vi "AK Komm.vi"(6 "Aktionen":T2=enum."initialisieren", 11 "Daten":string[](array[string])) -> (0 "Verfügbare Gase":string[][](array[string]), 1 "Empfangsdaten":string[](array[string]), 2 "Error":T1, 3 "Status":string, 4 "Störung Kommunikation":bool, 5 "Konzentration":sgl, 7 "Betriebsart":string)   [LabVIEW 2020, in "Linearisierung v2.lvlib" / "Gasteiler.lvlib" / "AK Komm Gasteiler.lvlib"]
uses:
  AK Komm Gasteiler.lvlib
  Aktionen AK Komm.ctl
  Gasteiler Fehler.ctl
  Aktionen FGV Gasteiler Daten.ctl
  Gasteiler Type.ctl
  Gasteiler.lvlib
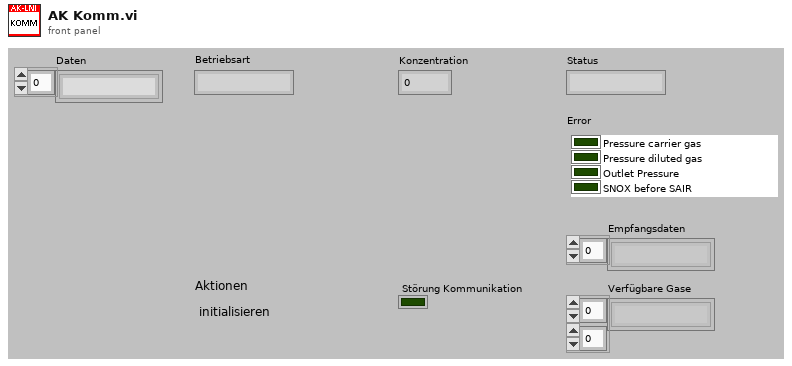
[diagram p1: front panel]
types:
  T1 = typedef "Linearisierung v2.lvlib/Gasteiler.lvlib/Gasteiler Fehler.ctl" = cluster{"Pressure carrier gas":bool, "Pressure diluted gas":bool, "Outlet Pressure":bool, "SNOX before SAIR":bool}
  T2 = typedef "Linearisierung v2.lvlib/Gasteiler.lvlib/AK Komm Gasteiler.lvlib/Aktionen AK Komm.ctl" = enum16{"lesen", "initialisieren", "beenden", "Status", "SMAN", "SREM", "STBY", "ASTF", "ASTZ", "SLST", "AGAT", "EGAK", "AGAK", "AKAK", "ADRU", "SKOP", "SVSA", "SVSZ", "SONO", "SAIR", "SNOX", "ANOX", "SSPL", "SRUC", "SLIN", "ALST", "ETYP", "SVIO", "LCYL", "CCYL", "DCYL", "SCYL", "GCYL", "DRGV", "DRDC"}
  T3 = typedef "Linearisierung v2.lvlib/Gasteiler.lvlib/Gasteiler Type.ctl" = enum16{"LNI Digital", "LNI Analoge", "AVL GDU ", "Horiba GDC", "HovaCal"}
  T4 = typedef "Linearisierung v2.lvlib/Gasteiler.lvlib/Aktionen FGV Gasteiler Daten.ctl" = enum16{"lesen", "Gasteiler Daten", "Seriellen Param.", "MB-Endwert", "laden", "speichern", "Anforderung", "TCP", "Aufzeichnung Start"}
  T5 = cluster{"Aktive":bool, "IP-Adresse":string, "Port":u16}
  T6 = typedef "Linearisierung v2.lvlib/GasteilerType.ctl" = u16
  T7 = typedef "AK-Schnittstelle.lvlib/AK Seriell.lvlib/Serielle Parameter.ctl" = cluster{"VISA resource name":refnum<visa-resource-name>, "baud rate":u32, "data bits":u16, "parity":u16, "stop bits":u16, "flow control":u16}
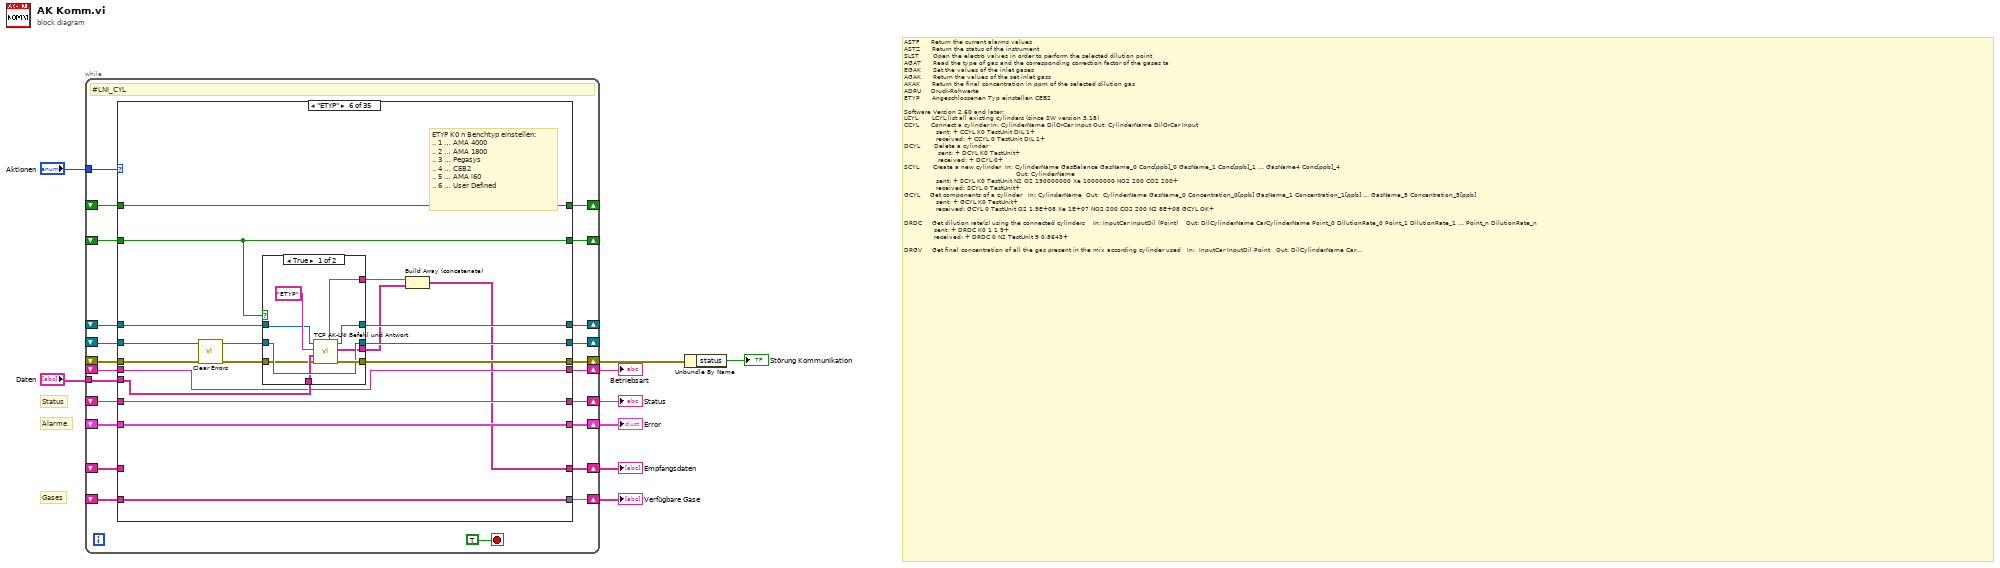
[diagram p0: block diagram]
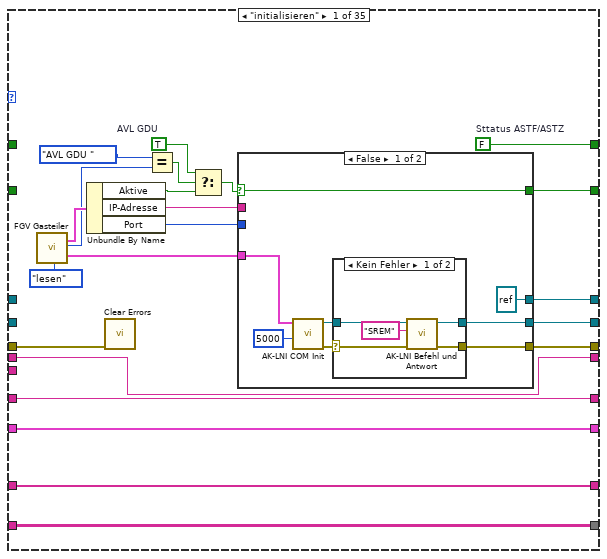
[diagram p2: hidden frame]
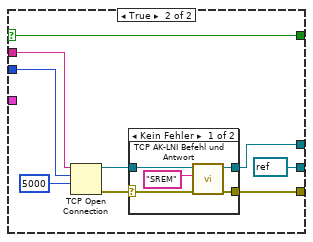
[diagram p4: hidden frame]
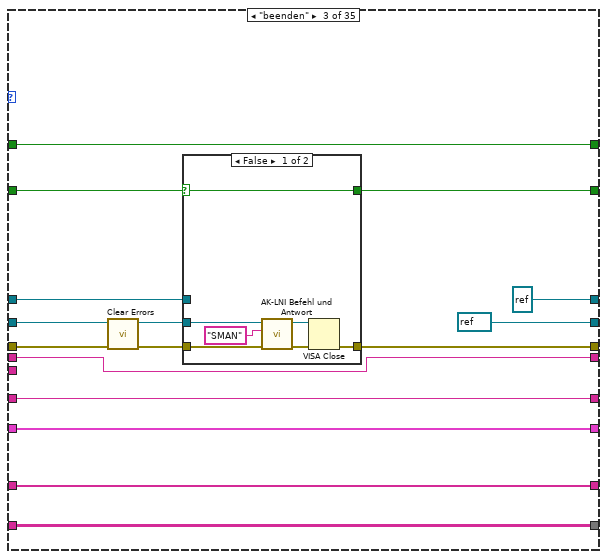
[diagram p7: hidden frame]
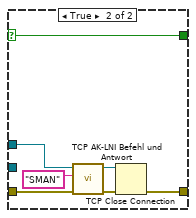
[diagram p8: hidden frame]
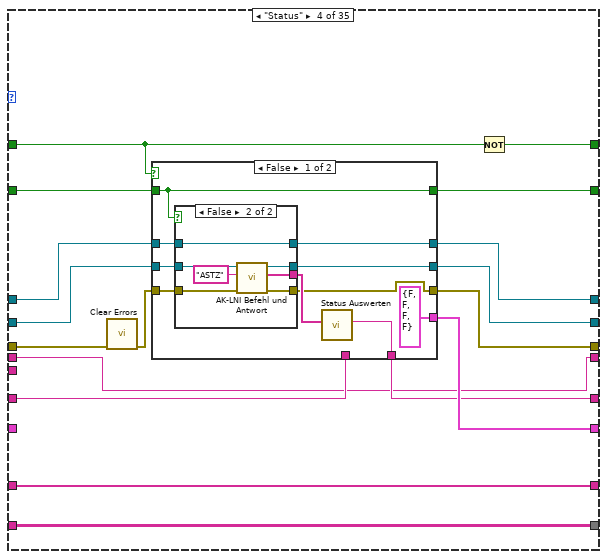
[diagram p9: hidden frame]
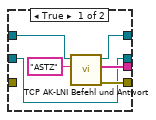
[diagram p10: hidden frame]
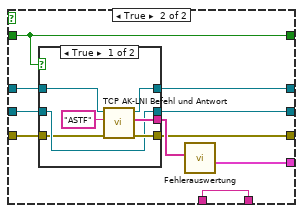
[diagram p11: hidden frame]
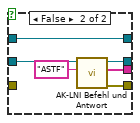
[diagram p12: hidden frame]
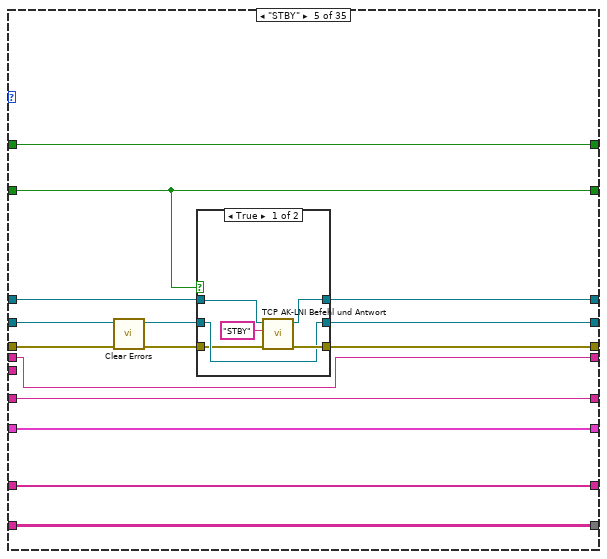
[diagram p13: hidden frame]
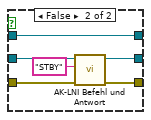
[diagram p14: hidden frame]
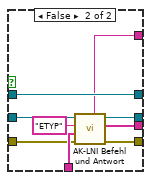
[diagram p15: hidden frame]
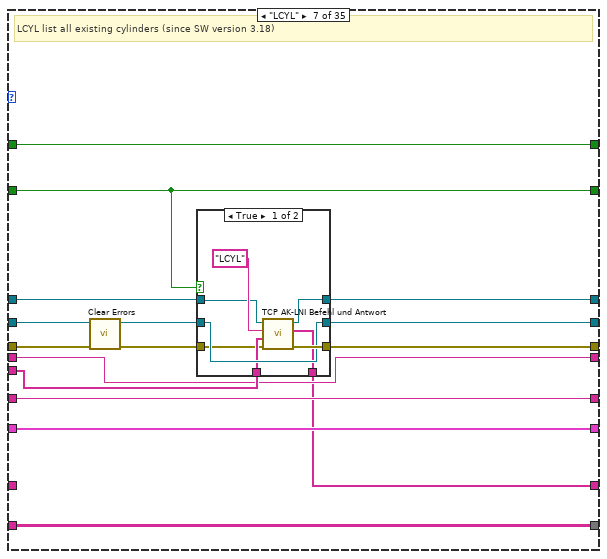
[diagram p16: hidden frame]
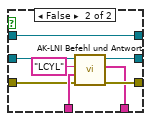
[diagram p17: hidden frame]
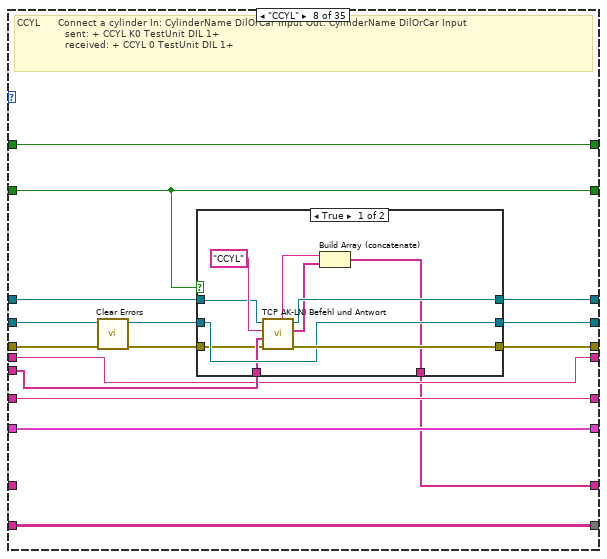
[diagram p18: hidden frame]
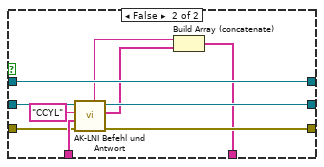
[diagram p19: hidden frame]
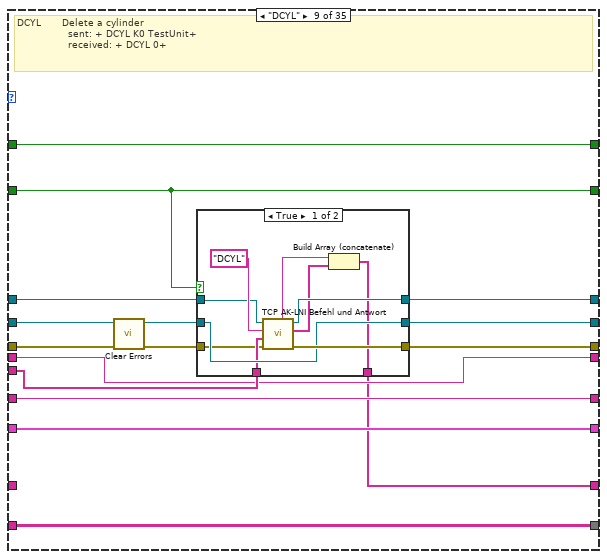
[diagram p20: hidden frame]
diagram:
  # "ASTF      Return the current alarms values\nASTZ      Return the status of the instrument \nSLST       Open the electro valves in order to perform the selected dilution point \nAGAT      Read the type of gas and the corresponding correction factor of the gases ta \nEGAK      Set the values of the inlet gases \nAGAK      Return the values of the set inlet gass \nAKAK      Return the final concentration in ppm of the selected dilution gas \nADRU     Druck-Rohwerte\nETYP      Angeschlossenen Typ einstellen CEB2\n\nSoftware Version 2.60 and later:\nLCYL       LCYL list all existing cylinders (since SW version 3.18)\nCCYL      Connect a cylinder In: CylinderName DilOrCar Input Out: CylinderName DilOrCar Input\n                sent: + CCYL K0 TestUnit DIL 1+\n                received: + CCYL 0 TestUnit DIL 1+\nDCYL       Delete a cylinder\n                 sent: + DCYL K0 TestUnit+\n                 received: + DCYL 0+\nSCYL       Create a new cylinder  In: CylinderName GasBalance GasName_0 Conc[ppb]_0 GasName_1 Conc[ppb]_1 … GasName4 Conc[ppb]_4\n                                                        Out: CylinderName\n                sent: + SCYL K0 TestUnit N2 O2 190000000 Xe 10000000 NO2 200 CO2 200+\n                received: SCYL 0 TestUnit+\nGCYL     Get components of a cylinder   In: CylinderName  Out:  CylinderName GasName_0 Concentration_0[ppb] GasName_1 Concentration_1[ppb] … GasName_5 Concentration_5[ppb]\n                sent: + GCYL K0 TestUnit+\n                received: GCYL 0 TestUnit O2 1.9E+08 Xe 1E+07 NO2 200 CO2 200 N2 8E+08 GCYL OK+\n\nDRDC     Get dilution rate(s) using the connected cylinders    In: InputCar InputDil (Point)    Out: DilCylinderName CarCylinderName Point_0 DilutionRate_0 Point_1 DilutionRate_1 … Point_n DilutionRate_n\n               sent: + DRDC K0 1 1 9+\n               received: + DRDC 0 N2 TestUnit 9 0.8643+\n\nDRGV     Get final concentration of all the gas present in the mix according cylinder used   In:  InputCar InputDil Point   Out: DilCylinderName CarCylinderName Point GasName_0 Concentration_0 GasName_1 Concentration_1 … GasName_n Concentration_n\n               sent: + DRGV K0 1 1 9+\n               received: + DRGV 0 N2 TestUnit 9 CO2 1.729 N2 9.983E+08 NO2 1.729 O2 1.642E+06 Xe 8.643E+04+ \n\nSKOP      Activate NOx converter tester \nSVSA      Open functions for the NOX converter tester \nSVSZ      Close functions for the NOX converter tester\nSONO     Open or close the valves in order to perform the NO phase\nSAIR       Open or close the valves in order to perform the Air phase of the NOx converter tester\nSNOX      Set the ozone in order to generate NO2 phase of the NOX converter tester (SONO and SAIR must have been sent previously)\nANOX      Read the set ozone value \n\n\n\nFür AVL\n\nSLIN        Um SLST senden zu können muss vorher SLIN gesendet werden\nALST        Abfrage Teilerstufe in %\n\nSVIO       Select the desired diluted inlet (if the option is installed). sent: + SVIO K0 13+ received: + SVIO 0"
  # "Gases"
  # "Status"
  # "Alarme"
  n1 = while {
    tunnel: "Aktionen" -> [w31]
    shift-right: [w30] -> _
    shift-left: _ -> [w29]
    shift-right: [w28] -> w4
    shift-left: _ -> [w27]
    shift-right: [w25] -> w7
    shift-left: _ -> [w26]
    tunnel: "Daten" -> [w24]
    shift-right: [w23] -> w5
    shift-left: _ -> [w22]
    shift-right: [w21] -> w6
    shift-left: _ -> [w20]
    shift-right: [w19] -> w3
    shift-left: _ -> [w18]
    shift-right: [w17] -> _
    shift-left: _ -> [w14]
    shift-right: [w16] -> _
    shift-left: _ -> [w15]
    shift-right: [w13] -> _
    shift-left: _ -> [w12]
    shift-right: [w11] -> w1
    shift-left: _ -> [w10]
    stop <- TRUE stop-if-true
    # "#LNI_CYL"
    n2 = case shown="\"ETYP\"" w31 {
      tunnel: [w49 w94 refnum<visa-resource-name> refnum ("VISA resource name") w140 w200 w229 w262 w293 w328 w363 w398 w433 w468 w504 w536 w567 w596 w626 w657 w694 w729 w767 w802 w834 w868 w899 w930 w963 w996 w1032 w1067 w1102 w1137 w1172 w1209] -> w30
      tunnel: w29 -> [_ w94 w104 w141 w201 w230 w263 w294 w329 w364 w399 w434 w469 w505 w537 w568 w597 w627 w658 w695 w730 w768 w803 w835 w869 w900 w931 w964 w997 w1033 w1068 w1103 w1138 w1173 w1210]
      tunnel: [w54 w95 w109 w131 w199 w228 w261 w292 w327 w362 w397 w432 w467 w503 w535 w561 w595 w625 w656 w693 w728 w766 w801 w833 w867 w898 w929 w962 w995 w1031 w1066 w1101 w1136 w1171 w1208] -> w28
      tunnel: w27 -> [w54 w95 w109 _ w199 w228 w261 w292 w327 w362 w397 w432 w467 w503 w535 _ w595 w625 w656 w693 w728 w766 w801 w833 w867 w898 w929 w962 w995 w1031 w1066 w1101 w1136 w1171 w1208]
      tunnel: w26 -> [w53 w92 w108 w129 w198 w227 w260 w291 w326 w361 w396 w431 w466 w502 w534 w565 _ _ w654 w691 w726 w764 w799 w832 w865 w896 w927 w960 w993 w1029 w1064 w1099 w1134 w1169 w1206]
      tunnel: [w53 w92 w108 w130 w198 w227 w260 w291 w326 w361 w396 w431 w466 w502 w534 w565 w593 w624 w654 w691 w726 w764 w799 w832 w865 w896 w927 w960 w993 w1029 w1064 w1099 w1134 w1169 w1206] -> w25
      tunnel: w24 -> [_ _ _ _ _ w219 w252 w283 w318 w353 w388 w423 w458 _ _ _ _ _ w655 w692 w727 w765 w800 _ w866 w897 w928 w961 w994 w1030 w1065 w1100 w1135 w1170 w1207]
      tunnel: [w51 w91 w106 w138 w196 w226 w259 w290 w325 w360 w395 w430 w465 w501 w533 w563 w591 w623 w653 w690 w725 w758 w798 w831 w864 w895 w926 w959 w992 w1028 w1063 w1098 w1133 w1168 w1205] -> w23
      tunnel: w22 -> [w51 w91 w106 w138 w196 w226 w259 w290 w325 w360 w395 w430 w465 w501 w533 w563 w591 w623 w653 w690 w725 _ w798 w831 w864 w895 w926 w959 w992 w1028 w1063 w1098 w1133 w1168 w1205]
      tunnel: [w52 w93 w107 w139 w197 w215 w250 w281 w316 w351 w386 w421 w456 w491 w523 w564 w592 w613 w645 w680 w715 w750 w787 w830 w856 w892 w918 w949 w984 w1019 w1053 w1088 w1123 w1158 w1193] -> w21
      tunnel: w20 -> [w52 w93 w107 w139 w197 _ _ _ _ _ _ _ _ _ _ w564 w592 _ _ _ _ _ _ _ _ _ _ _ _ _ _ _ _ _ _]
      tunnel: [w48 w90 w102 w137 w195 w225 w258 w289 w324 w359 w394 w429 w464 w500 w532 w562 w590 w622 w652 w689 w724 w761 w797 w829 w858 w894 w925 w958 w991 w1027 w1062 w1097 w1132 w1167 w1200] -> w19
      tunnel: w18 -> [w50 w90 w105 w136 w194 w224 w257 w288 w323 w358 w393 w428 w463 w499 w531 w560 w589 w621 w651 w688 w723 w760 w796 w828 w857 w893 w924 w957 w990 w1018 w1061 w1096 w1131 w1166 w1199]
      tunnel: [w44 w89 w101 w132 w193 w223 w256 w287 w322 w357 w392 w427 w462 w498 w530 w559 w588 w620 w650 w685 w722 w757 w795 w827 w855 w891 w923 w956 w989 w1026 w1060 w1095 w1130 w1165 w1198] -> w17
      tunnel: [w41 w88 refnum<k5> refnum ("Verbindungs-ID") w133 w191 w221 w254 w285 w320 w355 w390 w425 w460 w496 w528 w557 w586 w618 w648 w686 w720 w755 w793 w825 w853 w889 w921 w954 w987 w1024 w1058 w1093 w1128 w1163 w1196] -> w16
      tunnel: w15 -> [_ w88 w100 w134 w192 w222 w255 w286 w321 w356 w391 w426 w461 w497 w529 w558 w587 w619 w649 w687 w721 w756 w794 w826 w854 w890 w922 w955 w988 w1025 w1059 w1094 w1129 w1164 w1197]
      tunnel: w14 -> [_ w89 w103 w135 w193 w223 w256 w287 w322 w357 w392 w427 w462 w498 w530 w559 w588 w620 w650 w685 w722 w757 w795 w827 w855 w891 w923 w956 w989 w1026 w1060 w1095 w1130 w1165 w1198]
      tunnel: [w40 w87 w98 w127 w190 w220 w253 w284 w319 w354 w389 w424 w459 w495 w527 w556 w585 w617 w647 w684 w719 w754 w792 w824 w852 w888 w920 w953 w986 w1023 w1057 w1092 w1127 w1162 w1195] -> w13
      tunnel: w12 -> [_ w87 w98 w128 w190 w220 w253 w284 w319 w354 w389 w424 w459 w495 w527 w556 w585 w617 w647 w684 w719 w754 w792 w824 w852 w888 w920 w953 w986 w1023 w1057 w1092 w1127 w1162 w1195]
      tunnel: [w33 w86 w97 w126 w189 w218 w251 w282 w317 w352 w387 w422 w457 w494 w526 w555 w584 w616 w646 w683 w718 w753 w791 w823 w851 w887 w919 w952 w985 w1022 w1056 w1091 w1126 w1161 w1194] -> w11
      tunnel: w10 -> [w33 w86 w97 w126 w189 w218 w251 w282 w317 w352 w387 w422 w457 w494 w526 w555 _ w616 w646 w683 w718 w753 w791 w823 w851 w887 w919 w952 w985 w1022 w1056 w1091 w1126 w1161 w1194]
      frame "initialisieren" {
        w35 = TRUE  # AVL GDU
        w40 = FALSE  # Sttatus ASTF/ASTZ
        n3 = call "FGV Gasteiler.vi"("Aktionen"=Aktionen_FGV_Gasteiler_Daten."lesen") -> ("TCP"=w45:T5, "Gasteiler Type"=w39:T6, "Serielle Parameter"=w46:T7)  [unwired: 11 in, 5 out]
        n4 = Unbundle By Name(w45) -> ("Aktive"=w36:bool, "IP-Adresse"=w43:string, "Port"=w42:u16)
        n5 = call <vilib>:"Clear Errors.vi"("error in (no error)"=w50) -> ()  [unwired: 5 in, 2 out]
        n6 = Equal?(x=Gasteiler_Type."AVL GDU ", y=w39) -> (x = y?=w37:bool)
        n7 = Select(t=w35, s=w37, f=w36) -> (s? t:f=w34:bool)
        n8 = case shown="False" w34 {
          selector: w34 -> [w55 w78]
          tunnel: [w60 refnum<visa-resource-name> refnum ("VISA resource name")] -> w49
          tunnel: [w58 w73] -> w48
          tunnel: w46 -> [w57 _]
          tunnel: [w55 w78] -> w44
          tunnel: w43 -> [_ w76]
          tunnel: w42 -> [_ w75]
          tunnel: [refnum<k5> refnum ("connection ID") w70] -> w41
          frame False {
            n9 = call "AK-LNI COM Init.vi"("TimeOut (ms)"=u32 5000, "Schnittstelle"=w57) -> ("error out"=w59:errorcluster, "VISA resource name"=w61:refnum<visa-resource-name>)  [unwired: 8 in]
            n10 = case shown="Kein Fehler" w59 {
              selector: w59 -> [w64 w68]
              tunnel: w61 -> [w66 w69]
              tunnel: [w65 w69] -> w60
              tunnel: [w63 w68] -> w58
              frame No Error {
                n11 = call "AK-LNI Befehl und Antwort.vi"("Fehler (Eingang)"=w64, "Befehl (4 Zeichen)"="SREM", "VISA resource name"=w66) -> ("Fehler (Ausgang)"=w63:errorcluster, "VISA resource name out"=w65:refnum<visa-resource-name>)  [unwired: 3 in, 4 out]
              }
              frame Error {
              }
            }
          }
          frame True {
            n12 = TCP Open Connection(address=w76, remote port or service name=w75, timeout ms (60000)=5000 ("Timeout in ms (60000)")) -> (connection ID=w72:refnum<k5>, error out=w71:errorcluster)  [unwired: 2 in]
            n13 = case shown="Kein Fehler" w71 {
              selector: w71 -> [w79 w85]
              tunnel: [w83 w85] -> w73
              tunnel: w72 -> [w82 w84]
              tunnel: [w80 w84] -> w70
              frame No Error {
                n14 = call "TCP AK-LNI Befehl und Antwort.vi"("Fehler (Eingang)"=w79, "Befehl (4 Zeichen)"="SREM", "Verbindungs-ID"=w82) -> ("Fehler (Ausgang)"=w83:errorcluster, "Verbindungs-ID"=w80:refnum<k5>)  [unwired: 3 in, 4 out]
              }
              frame Error {
              }
            }
          }
        }
      }
      frame "lesen", Default {
      }
      frame "beenden" {
        n15 = call <vilib>:"Clear Errors.vi"("error in (no error)"=w105) -> ("error out"=w96:errorcluster)  [unwired: 5 in, 1 out]
        n16 = case shown="False" w103 {
          selector: w103 -> [w113 w124]
          tunnel: w104 -> [w117 _]
          tunnel: [w114 w119] -> w102
          tunnel: [w113 w124] -> w101
          tunnel: w100 -> [_ w123]
          tunnel: w96 -> [w111 w118]
          frame False {
            n17 = call "AK-LNI Befehl und Antwort.vi"("Fehler (Eingang)"=w111, "Befehl (4 Zeichen)"="SMAN", "VISA resource name"=w117) -> ("Fehler (Ausgang)"=w112:errorcluster, "VISA resource name out"=w115:refnum<visa-resource-name>)  [unwired: 3 in, 4 out]
            n18 = VISA Close(VISA resource name=w115, error in (no error)=w112) -> (error out=w114:errorcluster)
          }
          frame True {
            n19 = call "TCP AK-LNI Befehl und Antwort.vi"("Fehler (Eingang)"=w118, "Befehl (4 Zeichen)"="SMAN", "Verbindungs-ID"=w123) -> ("Fehler (Ausgang)"=w121:errorcluster, "Verbindungs-ID"=w120:refnum<k5>)  [unwired: 3 in, 4 out]
            n20 = TCP Close Connection(connection ID=w120, error in (no error)=w121) -> (error out=w119:errorcluster)  [unwired: 1 in, 1 out]
          }
        }
      }
      frame "Status" {
        n21 = call <vilib>:"Clear Errors.vi"("error in (no error)"=w136) -> ("error out"=w125:errorcluster)  [unwired: 5 in, 1 out]
        n22 = case shown="False" w128 {
          tunnel: w141 -> [w144 w174]
          tunnel: [w147 w173] -> w140
          tunnel: [w148 w171] -> w137
          tunnel: [T1 {"Pressure carrier gas"=FALSE, "Pressure diluted gas"=FALSE, "Outlet Pressure"=FALSE, "SNOX before SAIR"=FALSE} ("Error") w170] -> w131
          tunnel: w135 -> [w143 w167]
          tunnel: w134 -> [w145 w169]
          tunnel: [w146 w168] -> w133
          tunnel: [w143 w167] -> w132
          tunnel: [w150 w166] -> w130
          tunnel: w129 -> [_ w166]
          tunnel: w125 -> [w142 w165]
          frame False {
            n23 = case shown="False" w143 {
              tunnel: w144 -> [w154 w164]
              tunnel: [w154 w162] -> w147
              tunnel: [w156 w161] -> w151
              tunnel: [w155 w160] -> w148
              tunnel: w145 -> [w153 w159]
              tunnel: [w152 w159] -> w146
              tunnel: w142 -> [_ w158]
              frame True {
                n24 = call "TCP AK-LNI Befehl und Antwort.vi"("Befehl (4 Zeichen)"="ASTZ", "Verbindungs-ID"=w153) -> ("Fehler (Ausgang)"=w155:errorcluster, "Empfangsdaten"=w156:string[], "Verbindungs-ID"=w152:refnum<k5>)  [unwired: 4 in, 3 out]
              }
              frame False {
                n25 = call "AK-LNI Befehl und Antwort.vi"("Fehler (Eingang)"=w158, "Befehl (4 Zeichen)"="ASTZ", "VISA resource name"=w164) -> ("Fehler (Ausgang)"=w160:errorcluster, "Empfangsdaten"=w161:string[], "VISA resource name out"=w162:refnum<visa-resource-name>)  [unwired: 3 in, 3 out]
              }
            }
            n26 = call "Status Auswerten.vi"("Empfangsdaten"=w151) -> ("Status"=w150:string)  [unwired: 9 in, 1 out]
          }
          frame True {
            n27 = case shown="True" w167 {
              tunnel: w174 -> [w178 w187]
              tunnel: [w178 w185] -> w173
              tunnel: [w180 w184] -> w172
              tunnel: [w179 w183] -> w171
              tunnel: w169 -> [w177 w182]
              tunnel: [w176 w182] -> w168
              tunnel: w165 -> [w175 _]
              frame True {
                n28 = call "TCP AK-LNI Befehl und Antwort.vi"("Fehler (Eingang)"=w175, "Befehl (4 Zeichen)"="ASTF", "Verbindungs-ID"=w177) -> ("Fehler (Ausgang)"=w179:errorcluster, "Empfangsdaten"=w180:string[], "Verbindungs-ID"=w176:refnum<k5>)  [unwired: 3 in, 3 out]
              }
              frame False {
                n29 = call "AK-LNI Befehl und Antwort.vi"("Befehl (4 Zeichen)"="ASTF", "VISA resource name"=w187) -> ("Fehler (Ausgang)"=w183:errorcluster, "Empfangsdaten"=w184:string[], "VISA resource name out"=w185:refnum<visa-resource-name>)  [unwired: 4 in, 3 out]
              }
            }
            n30 = call "Fehlerauswertung.vi"("Empfangsdaten"=w172) -> ("Error"=w170:T1)  [unwired: 9 in, 1 out]
          }
        }
        n31 = Not(x=w128) -> (.not. x?=w127:bool)
      }
      frame "STBY" {
        n32 = call <vilib>:"Clear Errors.vi"("error in (no error)"=w194) -> ("error out"=w188:errorcluster)  [unwired: 5 in, 1 out]
        n33 = case shown="True" w193 {
          tunnel: w201 -> [w204 w213]
          tunnel: [w204 w211] -> w200
          tunnel: [w206 w210] -> w195
          tunnel: w192 -> [w205 w209]
          tunnel: [w203 w209] -> w191
          tunnel: w188 -> [w202 w208]
          frame True {
            n34 = call "TCP AK-LNI Befehl und Antwort.vi"("Fehler (Eingang)"=w202, "Befehl (4 Zeichen)"="STBY", "Verbindungs-ID"=w205) -> ("Fehler (Ausgang)"=w206:errorcluster, "Verbindungs-ID"=w203:refnum<k5>)  [unwired: 3 in, 4 out]
          }
          frame False {
            n35 = call "AK-LNI Befehl und Antwort.vi"("Fehler (Eingang)"=w208, "Befehl (4 Zeichen)"="STBY", "VISA resource name"=w213) -> ("Fehler (Ausgang)"=w210:errorcluster, "VISA resource name out"=w211:refnum<visa-resource-name>)  [unwired: 3 in, 4 out]
          }
        }
      }
      frame "ETYP" {
        # "ETYP K0 n Benchtyp einstellen:\n.. 1 … AMA 4000\n.. 2 … AMA 1800\n.. 3 … Pegasys\n.. 4 … CEB2\n.. 5 … AMA i60\n.. 6 … User Defined"
        n36 = call <vilib>:"Clear Errors.vi"("error in (no error)"=w224) -> ("error out"=w214:errorcluster)  [unwired: 5 in, 1 out]
        n37 = case shown="True" w223 {
          tunnel: w230 -> [w236 w248]
          tunnel: [w236 w246] -> w229
          tunnel: [w238 w245] -> w225
          tunnel: w222 -> [w237 w244]
          tunnel: [w235 w244] -> w221
          tunnel: w219 -> [w234 w243]
          tunnel: [w233 w242] -> w217
          tunnel: [w232 w241] -> w216
          tunnel: w214 -> [w231 w240]
          frame True {
            n38 = call "TCP AK-LNI Befehl und Antwort.vi"("Fehler (Eingang)"=w231, "Sendedaten"=w234, "Befehl (4 Zeichen)"="ETYP", "Verbindungs-ID"=w237) -> ("Fehler (Ausgang)"=w238:errorcluster, "Empfangsdaten"=w233:string[], "Verbindungs-ID"=w235:refnum<k5>, "Befehl (Antwort)"=w232:string)  [unwired: 2 in, 2 out]
          }
          frame False {
            n39 = call "AK-LNI Befehl und Antwort.vi"("Fehler (Eingang)"=w240, "Sendedaten"=w243, "Befehl (4 Zeichen)"="ETYP", "VISA resource name"=w248) -> ("Fehler (Ausgang)"=w245:errorcluster, "Empfangsdaten"=w242:string[], "VISA resource name out"=w246:refnum<visa-resource-name>, "Befehl (Antwort)"=w241:string)  [unwired: 2 in, 2 out]
          }
        }
        n40 = Build Array (concatenate)(w216, w217) -> (w215:string[])
      }
      frame "LCYL" {
        # "LCYL list all existing cylinders (since SW version 3.18)"
        n41 = call <vilib>:"Clear Errors.vi"("error in (no error)"=w257) -> ("error out"=w249:errorcluster)  [unwired: 5 in, 1 out]
        n42 = case shown="True" w256 {
          tunnel: w263 -> [w268 w279]
          tunnel: [w268 w277] -> w262
          tunnel: [w270 w276] -> w258
          tunnel: w255 -> [w269 w275]
          tunnel: [w267 w275] -> w254
          tunnel: w252 -> [w266 w274]
          tunnel: [w265 w273] -> w250
          tunnel: w249 -> [w264 w272]
          frame True {
            n43 = call "TCP AK-LNI Befehl und Antwort.vi"("Fehler (Eingang)"=w264, "Sendedaten"=w266, "Befehl (4 Zeichen)"="LCYL", "Verbindungs-ID"=w269) -> ("Fehler (Ausgang)"=w270:errorcluster, "Empfangsdaten"=w265:string[], "Verbindungs-ID"=w267:refnum<k5>)  [unwired: 2 in, 3 out]
          }
          frame False {
            n44 = call "AK-LNI Befehl und Antwort.vi"("Fehler (Eingang)"=w272, "Sendedaten"=w274, "Befehl (4 Zeichen)"="LCYL", "VISA resource name"=w279) -> ("Fehler (Ausgang)"=w276:errorcluster, "Empfangsdaten"=w273:string[], "VISA resource name out"=w277:refnum<visa-resource-name>)  [unwired: 2 in, 3 out]
          }
        }
      }
      frame "CCYL" {
        # "CCYL      Connect a cylinder In: CylinderName DilOrCar Input Out: CylinderName DilOrCar Input\n                sent: + CCYL K0 TestUnit DIL 1+\n                received: + CCYL 0 TestUnit DIL 1+"
        n45 = call <vilib>:"Clear Errors.vi"("error in (no error)"=w288) -> ("error out"=w280:errorcluster)  [unwired: 5 in, 1 out]
        n46 = case shown="True" w287 {
          tunnel: w294 -> [w301 w314]
          tunnel: [w301 w312] -> w293
          tunnel: [w303 w311] -> w289
          tunnel: w286 -> [w302 w310]
          tunnel: [w300 w310] -> w285
          tunnel: w283 -> [w299 w309]
          tunnel: [w296 w306] -> w281
          tunnel: w280 -> [w295 w305]
          frame True {
            n47 = call "TCP AK-LNI Befehl und Antwort.vi"("Fehler (Eingang)"=w295, "Sendedaten"=w299, "Befehl (4 Zeichen)"="CCYL", "Verbindungs-ID"=w302) -> ("Fehler (Ausgang)"=w303:errorcluster, "Empfangsdaten"=w297:string[], "Verbindungs-ID"=w300:refnum<k5>, "Befehl (Antwort)"=w298:string)  [unwired: 2 in, 2 out]
            n48 = Build Array (concatenate)(w298, w297) -> (w296:string[])
          }
          frame False {
            n49 = call "AK-LNI Befehl und Antwort.vi"("Fehler (Eingang)"=w305, "Sendedaten"=w309, "Befehl (4 Zeichen)"="CCYL", "VISA resource name"=w314) -> ("Fehler (Ausgang)"=w311:errorcluster, "Empfangsdaten"=w307:string[], "VISA resource name out"=w312:refnum<visa-resource-name>, "Befehl (Antwort)"=w308:string)  [unwired: 2 in, 2 out]
            n50 = Build Array (concatenate)(w308, w307) -> (w306:string[])
          }
        }
      }
      frame "DCYL" {
        # "DCYL       Delete a cylinder\n                 sent: + DCYL K0 TestUnit+\n                 received: + DCYL 0+"
        n51 = call <vilib>:"Clear Errors.vi"("error in (no error)"=w323) -> ("error out"=w315:errorcluster)  [unwired: 5 in, 1 out]
        n52 = case shown="True" w322 {
          tunnel: w329 -> [w336 w349]
          tunnel: [w336 w347] -> w328
          tunnel: [w338 w346] -> w324
          tunnel: w321 -> [w337 w345]
          tunnel: [w335 w345] -> w320
          tunnel: w318 -> [w334 w344]
          tunnel: [w331 w341] -> w316
          tunnel: w315 -> [w330 w340]
          frame True {
            n53 = call "TCP AK-LNI Befehl und Antwort.vi"("Fehler (Eingang)"=w330, "Sendedaten"=w334, "Befehl (4 Zeichen)"="DCYL", "Verbindungs-ID"=w337) -> ("Fehler (Ausgang)"=w338:errorcluster, "Empfangsdaten"=w332:string[], "Verbindungs-ID"=w335:refnum<k5>, "Befehl (Antwort)"=w333:string)  [unwired: 2 in, 2 out]
            n54 = Build Array (concatenate)(w333, w332) -> (w331:string[])
          }
          frame False {
            n55 = call "AK-LNI Befehl und Antwort.vi"("Fehler (Eingang)"=w340, "Sendedaten"=w344, "Befehl (4 Zeichen)"="DCYL", "VISA resource name"=w349) -> ("Fehler (Ausgang)"=w346:errorcluster, "Empfangsdaten"=w342:string[], "VISA resource name out"=w347:refnum<visa-resource-name>, "Befehl (Antwort)"=w343:string)  [unwired: 2 in, 2 out]
            n56 = Build Array (concatenate)(w343, w342) -> (w341:string[])
          }
        }
      }
      frame "SCYL" {
        # "SCYL       Create a new cylinder  In: CylinderName GasBalance GasName_0 Conc[ppb]_0 GasName_1 Conc[ppb]_1 … GasName4 Conc[ppb]_4\n                                                        Out: CylinderName\n                sent: + SCYL K0 TestUnit N2 O2 190000000 Xe 10000000 NO2 200 CO2 200+\n                received: SCYL 0 TestUnit+"
        n57 = call <vilib>:"Clear Errors.vi"("error in (no error)"=w358) -> ("error out"=w350:errorcluster)  [unwired: 5 in, 1 out]
        n58 = case shown="True" w357 {
          tunnel: w364 -> [w371 w384]
          tunnel: [w371 w382] -> w363
          tunnel: [w373 w381] -> w359
          tunnel: w356 -> [w372 w380]
          tunnel: [w370 w380] -> w355
          tunnel: w353 -> [w369 w379]
          tunnel: [w366 w376] -> w351
          tunnel: w350 -> [w365 w375]
          frame True {
            n59 = call "TCP AK-LNI Befehl und Antwort.vi"("Fehler (Eingang)"=w365, "Sendedaten"=w369, "Befehl (4 Zeichen)"="SCYL", "Verbindungs-ID"=w372) -> ("Fehler (Ausgang)"=w373:errorcluster, "Empfangsdaten"=w367:string[], "Verbindungs-ID"=w370:refnum<k5>, "Befehl (Antwort)"=w368:string)  [unwired: 2 in, 2 out]
            n60 = Build Array (concatenate)(w368, w367) -> (w366:string[])
          }
          frame False {
            n61 = call "AK-LNI Befehl und Antwort.vi"("Fehler (Eingang)"=w375, "Sendedaten"=w379, "Befehl (4 Zeichen)"="SCYL", "VISA resource name"=w384) -> ("Fehler (Ausgang)"=w381:errorcluster, "Empfangsdaten"=w377:string[], "VISA resource name out"=w382:refnum<visa-resource-name>, "Befehl (Antwort)"=w378:string)  [unwired: 2 in, 2 out]
            n62 = Build Array (concatenate)(w378, w377) -> (w376:string[])
          }
        }
      }
      frame "GCYL" {
        # "GCYL     Get components of a cylinder   In: CylinderName  Out:  CylinderName GasName_0 Concentration_0[ppb] GasName_1 Concentration_1[ppb] … GasName_5 Concentration_5[ppb]\n                sent: + GCYL K0 TestUnit+\n                received: GCYL 0 TestUnit O2 1.9E+08 Xe 1E+07 NO2 200 CO2 200 N2 8E+08 GCYL OK+"
        n63 = call <vilib>:"Clear Errors.vi"("error in (no error)"=w393) -> ("error out"=w385:errorcluster)  [unwired: 5 in, 1 out]
        n64 = case shown="True" w392 {
          tunnel: w399 -> [w406 w419]
          tunnel: [w406 w417] -> w398
          tunnel: [w408 w416] -> w394
          tunnel: w391 -> [w407 w415]
          tunnel: [w405 w415] -> w390
          tunnel: w388 -> [w404 w414]
          tunnel: [w401 w411] -> w386
          tunnel: w385 -> [w400 w410]
          frame True {
            n65 = call "TCP AK-LNI Befehl und Antwort.vi"("Fehler (Eingang)"=w400, "Sendedaten"=w404, "Befehl (4 Zeichen)"="GCYL", "Verbindungs-ID"=w407) -> ("Fehler (Ausgang)"=w408:errorcluster, "Empfangsdaten"=w402:string[], "Verbindungs-ID"=w405:refnum<k5>, "Befehl (Antwort)"=w403:string)  [unwired: 2 in, 2 out]
            n66 = Build Array (concatenate)(w403, w402) -> (w401:string[])
          }
          frame False {
            n67 = call "AK-LNI Befehl und Antwort.vi"("Fehler (Eingang)"=w410, "Sendedaten"=w414, "Befehl (4 Zeichen)"="GCYL", "VISA resource name"=w419) -> ("Fehler (Ausgang)"=w416:errorcluster, "Empfangsdaten"=w412:string[], "VISA resource name out"=w417:refnum<visa-resource-name>, "Befehl (Antwort)"=w413:string)  [unwired: 2 in, 2 out]
            n68 = Build Array (concatenate)(w413, w412) -> (w411:string[])
          }
        }
      }
      frame "DRGV" {
        # "Get final concentration of all the gas present in the mix according cylinder used   In:  InputCar InputDil Point   Out: DilCylinderName CarCylinderName Point GasName_0 Concentration_0 GasName_1 Concentration_1 … GasName_n Concentration_n\n               sent: + DRGV K0 1 1 9+\n               received: + DRGV 0 N2 TestUnit 9 CO2 1.729 N2 9.983E+08 NO2 1.729 O2 1.642E+06 Xe 8.643E+04+"
        n69 = call <vilib>:"Clear Errors.vi"("error in (no error)"=w428) -> ("error out"=w420:errorcluster)  [unwired: 5 in, 1 out]
        n70 = case shown="True" w427 {
          tunnel: w434 -> [w441 w454]
          tunnel: [w441 w452] -> w433
          tunnel: [w443 w451] -> w429
          tunnel: w426 -> [w442 w450]
          tunnel: [w440 w450] -> w425
          tunnel: w423 -> [w439 w449]
          tunnel: [w436 w446] -> w421
          tunnel: w420 -> [w435 w445]
          frame True {
            n71 = call "TCP AK-LNI Befehl und Antwort.vi"("Fehler (Eingang)"=w435, "Sendedaten"=w439, "Befehl (4 Zeichen)"="DRGV", "Verbindungs-ID"=w442) -> ("Fehler (Ausgang)"=w443:errorcluster, "Empfangsdaten"=w437:string[], "Verbindungs-ID"=w440:refnum<k5>, "Befehl (Antwort)"=w438:string)  [unwired: 2 in, 2 out]
            n72 = Build Array (concatenate)(w438, w437) -> (w436:string[])
          }
          frame False {
            n73 = call "AK-LNI Befehl und Antwort.vi"("Fehler (Eingang)"=w445, "Sendedaten"=w449, "Befehl (4 Zeichen)"="DRGV", "VISA resource name"=w454) -> ("Fehler (Ausgang)"=w451:errorcluster, "Empfangsdaten"=w447:string[], "VISA resource name out"=w452:refnum<visa-resource-name>, "Befehl (Antwort)"=w448:string)  [unwired: 2 in, 2 out]
            n74 = Build Array (concatenate)(w448, w447) -> (w446:string[])
          }
        }
      }
      frame "DRDC" {
        # "Get dilution rate(s) using the connected cylinders    In: InputCar InputDil (Point)    Out: DilCylinderName CarCylinderName Point_0 DilutionRate_0 Point_1 DilutionRate_1 … Point_n DilutionRate_n\n               sent: + DRDC K0 1 1 9+\n               received: + DRDC 0 N2 TestUnit 9 0.8643+"
        n75 = call <vilib>:"Clear Errors.vi"("error in (no error)"=w463) -> ("error out"=w455:errorcluster)  [unwired: 5 in, 1 out]
        n76 = case shown="True" w462 {
          tunnel: w469 -> [w476 w489]
          tunnel: [w476 w487] -> w468
          tunnel: [w478 w486] -> w464
          tunnel: w461 -> [w477 w485]
          tunnel: [w475 w485] -> w460
          tunnel: w458 -> [w474 w484]
          tunnel: [w471 w481] -> w456
          tunnel: w455 -> [w470 w480]
          frame True {
            n77 = call "TCP AK-LNI Befehl und Antwort.vi"("Fehler (Eingang)"=w470, "Sendedaten"=w474, "Befehl (4 Zeichen)"="DRDC", "Verbindungs-ID"=w477) -> ("Fehler (Ausgang)"=w478:errorcluster, "Empfangsdaten"=w472:string[], "Verbindungs-ID"=w475:refnum<k5>, "Befehl (Antwort)"=w473:string)  [unwired: 2 in, 2 out]
            n78 = Build Array (concatenate)(w473, w472) -> (w471:string[])
          }
          frame False {
            n79 = call "AK-LNI Befehl und Antwort.vi"("Fehler (Eingang)"=w480, "Sendedaten"=w484, "Befehl (4 Zeichen)"="DRDC", "VISA resource name"=w489) -> ("Fehler (Ausgang)"=w486:errorcluster, "Empfangsdaten"=w482:string[], "VISA resource name out"=w487:refnum<visa-resource-name>, "Befehl (Antwort)"=w483:string)  [unwired: 2 in, 2 out]
            n80 = Build Array (concatenate)(w483, w482) -> (w481:string[])
          }
        }
      }
      frame "SMAN" {
        n81 = call <vilib>:"Clear Errors.vi"("error in (no error)"=w499) -> ("error out"=w490:errorcluster)  [unwired: 5 in, 1 out]
        n82 = case shown="False" w498 {
          tunnel: w505 -> [w511 w521]
          tunnel: [w511 w519] -> w504
          tunnel: [w512 w518] -> w500
          tunnel: w497 -> [w510 w517]
          tunnel: [w509 w517] -> w496
          tunnel: [w508 w516] -> w492
          tunnel: [w507 w515] -> w493
          tunnel: w490 -> [w506 w514]
          frame True {
            n83 = call "TCP AK-LNI Befehl und Antwort.vi"("Fehler (Eingang)"=w506, "Befehl (4 Zeichen)"="SMAN", "Verbindungs-ID"=w510) -> ("Fehler (Ausgang)"=w512:errorcluster, "Empfangsdaten"=w508:string[], "Verbindungs-ID"=w509:refnum<k5>, "Befehl (Antwort)"=w507:string)  [unwired: 3 in, 2 out]
          }
          frame False {
            n84 = call "AK-LNI Befehl und Antwort.vi"("Fehler (Eingang)"=w514, "Befehl (4 Zeichen)"="SMAN", "VISA resource name"=w521) -> ("Fehler (Ausgang)"=w518:errorcluster, "Empfangsdaten"=w516:string[], "VISA resource name out"=w519:refnum<visa-resource-name>, "Befehl (Antwort)"=w515:string)  [unwired: 3 in, 2 out]
          }
        }
        n85 = Build Array (concatenate)(w493, w492) -> (w491:string[])
      }
      frame "SREM" {
        n86 = call <vilib>:"Clear Errors.vi"("error in (no error)"=w531) -> ("error out"=w522:errorcluster)  [unwired: 5 in, 1 out]
        n87 = case shown="False" w530 {
          tunnel: w537 -> [w541 w553]
          tunnel: [w541 w551] -> w536
          tunnel: [w544 w550] -> w532
          tunnel: w529 -> [w543 w549]
          tunnel: [w542 w549] -> w528
          tunnel: [w540 w548] -> w524
          tunnel: [w539 w546] -> w525
          tunnel: w522 -> [w538 w547]
          frame True {
            n88 = call "TCP AK-LNI Befehl und Antwort.vi"("Fehler (Eingang)"=w538, "Befehl (4 Zeichen)"="SREM", "Verbindungs-ID"=w543) -> ("Fehler (Ausgang)"=w544:errorcluster, "Empfangsdaten"=w540:string[], "Verbindungs-ID"=w542:refnum<k5>, "Befehl (Antwort)"=w539:string)  [unwired: 3 in, 2 out]
          }
          frame False {
            n89 = call "AK-LNI Befehl und Antwort.vi"("Fehler (Eingang)"=w547, "Befehl (4 Zeichen)"="SREM", "VISA resource name"=w553) -> ("Fehler (Ausgang)"=w550:errorcluster, "Empfangsdaten"=w548:string[], "VISA resource name out"=w551:refnum<visa-resource-name>, "Befehl (Antwort)"=w546:string)  [unwired: 3 in, 2 out]
          }
        }
        n90 = Build Array (concatenate)(w525, w524) -> (w523:string[])
      }
      frame "ASTF" {
        # "Return the current alarms values\n\nBefehl:     ASTF K0\nAntwort:  ASTF ES X Y ... N\n\nAlarm Code: 0  if there are no alarms\n                     1  if the pressure of the carrier gas is out of range\n                     2  if the pressure of the diluted gas is out of range\n                     3  if the outlet pressure is out of range\n                     4  if the command SNOX have been sent before the SAIR command"
        n91 = call <vilib>:"Clear Errors.vi"("error in (no error)"=w560) -> ("error out"=w554:errorcluster)  [unwired: 5 in, 1 out]
        n92 = case shown="True" w559 {
          tunnel: w568 -> [w572 w582]
          tunnel: [w572 w580] -> w567
          tunnel: [w574 w579] -> w566
          tunnel: [w573 w578] -> w562
          tunnel: w558 -> [w571 w577]
          tunnel: [w570 w577] -> w557
          tunnel: w554 -> [w569 w576]
          frame True {
            n93 = call "TCP AK-LNI Befehl und Antwort.vi"("Fehler (Eingang)"=w569, "Befehl (4 Zeichen)"="ASTF", "Verbindungs-ID"=w571) -> ("Fehler (Ausgang)"=w573:errorcluster, "Empfangsdaten"=w574:string[], "Verbindungs-ID"=w570:refnum<k5>)  [unwired: 3 in, 3 out]
          }
          frame False {
            n94 = call "AK-LNI Befehl und Antwort.vi"("Fehler (Eingang)"=w576, "Befehl (4 Zeichen)"="ASTF", "VISA resource name"=w582) -> ("Fehler (Ausgang)"=w578:errorcluster, "Empfangsdaten"=w579:string[], "VISA resource name out"=w580:refnum<visa-resource-name>)  [unwired: 3 in, 3 out]
          }
        }
        n95 = call "Fehlerauswertung.vi"("Empfangsdaten"=w566) -> ("Error"=w561:T1)  [unwired: 9 in, 1 out]
      }
      frame "ASTZ" {
        # "Return the status of the instrument \n\nBefehl:     ASTZ K0\nAntwort:  ASTZ ES Stat1 Stat2\n\nStat1 = SREM oder SMAN\nStat2 = STBY\n             SLST Point\n             SSPL Phase\n             SRUC Phase\n             SAIR\n             SONO\n             SNOX O3_Value"
        n96 = call <vilib>:"Clear Errors.vi"("error in (no error)"=w589) -> ("error out"=w583:errorcluster)  [unwired: 5 in, 1 out]
        n97 = case shown="True" w588 {
          tunnel: w597 -> [w601 w611]
          tunnel: [w601 w609] -> w596
          tunnel: [w603 w608] -> w594
          tunnel: [w602 w607] -> w590
          tunnel: w587 -> [w600 w606]
          tunnel: [w599 w606] -> w586
          tunnel: w583 -> [w598 w605]
          frame True {
            n98 = call "TCP AK-LNI Befehl und Antwort.vi"("Fehler (Eingang)"=w598, "Befehl (4 Zeichen)"="ASTZ", "Verbindungs-ID"=w600) -> ("Fehler (Ausgang)"=w602:errorcluster, "Empfangsdaten"=w603:string[], "Verbindungs-ID"=w599:refnum<k5>)  [unwired: 3 in, 3 out]
          }
          frame False {
            n99 = call "AK-LNI Befehl und Antwort.vi"("Fehler (Eingang)"=w605, "Befehl (4 Zeichen)"="ASTZ", "VISA resource name"=w611) -> ("Fehler (Ausgang)"=w607:errorcluster, "Empfangsdaten"=w608:string[], "VISA resource name out"=w609:refnum<visa-resource-name>)  [unwired: 3 in, 3 out]
          }
        }
        n100 = call "Status Auswerten.vi"("Empfangsdaten"=w594) -> ("Status"=w593:string, "Betriebsart"=w584:string)  [unwired: 9 in]
      }
      frame "SLIN" {
        n101 = call <vilib>:"Clear Errors.vi"("error in (no error)"=w621) -> ("error out"=w612:errorcluster)  [unwired: 5 in, 1 out]
        n102 = case shown="False" w620 {
          tunnel: w627 -> [w632 w643]
          tunnel: [w632 w641] -> w626
          tunnel: [w634 w640] -> w614
          tunnel: [w633 w639] -> w622
          tunnel: w619 -> [w631 w638]
          tunnel: [w630 w638] -> w618
          tunnel: [w629 w637] -> w615
          tunnel: w612 -> [w628 w636]
          frame True {
            n103 = call "TCP AK-LNI Befehl und Antwort.vi"("Fehler (Eingang)"=w628, "Befehl (4 Zeichen)"="SLIN", "Verbindungs-ID"=w631) -> ("Fehler (Ausgang)"=w633:errorcluster, "Empfangsdaten"=w634:string[], "Verbindungs-ID"=w630:refnum<k5>, "Befehl (Antwort)"=w629:string)  [unwired: 3 in, 2 out]
          }
          frame False {
            n104 = call "AK-LNI Befehl und Antwort.vi"("Fehler (Eingang)"=w636, "Befehl (4 Zeichen)"="SLIN", "VISA resource name"=w643) -> ("Fehler (Ausgang)"=w639:errorcluster, "Empfangsdaten"=w640:string[], "VISA resource name out"=w641:refnum<visa-resource-name>, "Befehl (Antwort)"=w637:string)  [unwired: 3 in, 2 out]
          }
        }
        n105 = call "Status Auswerten.vi"("Empfangsdaten"=w614) -> ("Status"=w624:string)  [unwired: 9 in, 1 out]
        n106 = Build Array (concatenate)(w615, w614) -> (w613:string[])
      }
      frame "SLST" {
        # "Open the electro valves in order to perform the selected dilution point\n\nBefehl:     SLST K0 Arg\nAntwort:  SLST ES\n\nArg = dilution point"
        n107 = call <vilib>:"Clear Errors.vi"("error in (no error)"=w651) -> ("error out"=w644:errorcluster)  [unwired: 5 in, 1 out]
        n108 = case shown="False" w650 {
          tunnel: w658 -> [w665 w678]
          tunnel: [w665 w676] -> w657
          tunnel: w655 -> [w667 w675]
          tunnel: [w666 w674] -> w652
          tunnel: w649 -> [w664 w673]
          tunnel: [w663 w673] -> w648
          tunnel: [w660 w670] -> w645
          tunnel: w644 -> [w659 w669]
          frame True {
            n109 = call "TCP AK-LNI Befehl und Antwort.vi"("Fehler (Eingang)"=w659, "Sendedaten"=w667, "Befehl (4 Zeichen)"="SLST", "Verbindungs-ID"=w664) -> ("Fehler (Ausgang)"=w666:errorcluster, "Empfangsdaten"=w661:string[], "Verbindungs-ID"=w663:refnum<k5>, "Befehl (Antwort)"=w662:string)  [unwired: 2 in, 2 out]
            n110 = Build Array (concatenate)(w662, w661) -> (w660:string[])
          }
          frame False {
            n111 = call "AK-LNI Befehl und Antwort.vi"("Fehler (Eingang)"=w669, "Sendedaten"=w675, "Befehl (4 Zeichen)"="SLST", "VISA resource name"=w678) -> ("Fehler (Ausgang)"=w674:errorcluster, "Empfangsdaten"=w671:string[], "VISA resource name out"=w676:refnum<visa-resource-name>, "Befehl (Antwort)"=w672:string)  [unwired: 2 in, 2 out]
            n112 = Build Array (concatenate)(w672, w671) -> (w670:string[])
          }
        }
      }
      frame "SSPL" {
        # "Open the electro valves in order to perform a purge\n\nBefehl:     SSPL K0 \nAntwort:  SSPL ES"
        n113 = call <vilib>:"Clear Errors.vi"("error in (no error)"=w688) -> ("error out"=w679:errorcluster)  [unwired: 5 in, 1 out]
        n114 = case shown="True" w685 {
          tunnel: w695 -> [w701 w713]
          tunnel: [w701 w711] -> w694
          tunnel: w692 -> [w703 w710]
          tunnel: [w702 w709] -> w689
          tunnel: w687 -> [w700 w708]
          tunnel: [w699 w708] -> w686
          tunnel: [w698 w707] -> w681
          tunnel: [w697 w706] -> w682
          tunnel: w679 -> [w696 w705]
          frame True {
            n115 = call "TCP AK-LNI Befehl und Antwort.vi"("Fehler (Eingang)"=w696, "Sendedaten"=w703, "Befehl (4 Zeichen)"="SSPL", "Verbindungs-ID"=w700) -> ("Fehler (Ausgang)"=w702:errorcluster, "Empfangsdaten"=w698:string[], "Verbindungs-ID"=w699:refnum<k5>, "Befehl (Antwort)"=w697:string)  [unwired: 2 in, 2 out]
          }
          frame False {
            n116 = call "AK-LNI Befehl und Antwort.vi"("Fehler (Eingang)"=w705, "Sendedaten"=w710, "Befehl (4 Zeichen)"="SSPL", "VISA resource name"=w713) -> ("Fehler (Ausgang)"=w709:errorcluster, "Empfangsdaten"=w707:string[], "VISA resource name out"=w711:refnum<visa-resource-name>, "Befehl (Antwort)"=w706:string)  [unwired: 2 in, 2 out]
          }
        }
        n117 = Build Array (concatenate)(w682, w681) -> (w680:string[])
      }
      frame "SRUC" {
        # "Open the electro valves in order to perform a purge with the carrier gases\n\nBefehl:     SRUC K0 \nAntwort:  SRUC ES"
        n118 = call <vilib>:"Clear Errors.vi"("error in (no error)"=w723) -> ("error out"=w714:errorcluster)  [unwired: 5 in, 1 out]
        n119 = case shown="True" w722 {
          tunnel: w730 -> [w734 w748]
          tunnel: [w734 w746] -> w729
          tunnel: w727 -> [w738 w745]
          tunnel: [w737 w744] -> w724
          tunnel: w721 -> [w736 w743]
          tunnel: [w735 w743] -> w720
          tunnel: [w733 w742] -> w716
          tunnel: [w732 w741] -> w717
          tunnel: w714 -> [w731 w740]
          frame True {
            n120 = call "TCP AK-LNI Befehl und Antwort.vi"("Fehler (Eingang)"=w731, "Sendedaten"=w738, "Befehl (4 Zeichen)"="SRUC", "Verbindungs-ID"=w736) -> ("Fehler (Ausgang)"=w737:errorcluster, "Empfangsdaten"=w733:string[], "Verbindungs-ID"=w735:refnum<k5>, "Befehl (Antwort)"=w732:string)  [unwired: 2 in, 2 out]
          }
          frame False {
            n121 = call "AK-LNI Befehl und Antwort.vi"("Fehler (Eingang)"=w740, "Sendedaten"=w745, "Befehl (4 Zeichen)"="SRUC", "VISA resource name"=w748) -> ("Fehler (Ausgang)"=w744:errorcluster, "Empfangsdaten"=w742:string[], "VISA resource name out"=w746:refnum<visa-resource-name>, "Befehl (Antwort)"=w741:string)  [unwired: 2 in, 2 out]
          }
        }
        n122 = Build Array (concatenate)(w717, w716) -> (w715:string[])
      }
      frame "AGAT" {
        # "Read the type of gas and the corresponding correction factor of the gases table\n\nBefehl:    AGAT K0\nAntwort: AGAT ES Gas1 Cf1 Gas2 Cf2 ..."
        n123 = call <vilib>:"Clear Errors.vi"("error in (no error)"=w760) -> ("error out"=w749:errorcluster)  [unwired: 5 in, 1 out]
        n124 = case shown="False" w757 {
          tunnel: w768 -> [w771 w786]
          tunnel: [w771 w784] -> w767
          tunnel: w765 -> [w776 w783]
          tunnel: [w775 w782] -> w751
          tunnel: [w774 w781] -> w761
          tunnel: w756 -> [w773 w780]
          tunnel: [w772 w780] -> w755
          tunnel: [w770 w779] -> w752
          tunnel: w749 -> [w769 w778]
          frame True {
            n125 = call "TCP AK-LNI Befehl und Antwort.vi"("Fehler (Eingang)"=w769, "Sendedaten"=w776, "Befehl (4 Zeichen)"="AGAT", "Verbindungs-ID"=w773) -> ("Fehler (Ausgang)"=w774:errorcluster, "Empfangsdaten"=w775:string[], "Verbindungs-ID"=w772:refnum<k5>, "Befehl (Antwort)"=w770:string)  [unwired: 2 in, 2 out]
          }
          frame False {
            n126 = call "AK-LNI Befehl und Antwort.vi"("Fehler (Eingang)"=w778, "Sendedaten"=w783, "Befehl (4 Zeichen)"="AGAT", "VISA resource name"=w786) -> ("Fehler (Ausgang)"=w781:errorcluster, "Empfangsdaten"=w782:string[], "VISA resource name out"=w784:refnum<visa-resource-name>, "Befehl (Antwort)"=w779:string)  [unwired: 2 in, 2 out]
          }
        }
        n127 = Decimate 1D Array(w751) -> (w763:string[], w762:string[])
        n128 = Build Array (concatenate)(w752, w751) -> (w750:string[])
        n129 = Build Array(w763, w762) -> (w759:string[][])
        n130 = Transpose 2D Array(2D array=w759) -> (transposed array=w758:string[][])
      }
      frame "EGAK" {
        # "Set the values of the inlet gases\n\nBefehl:     EGAK K0 Gas1 Gas2 Arg\nAntwort:  EGAK K0\n\nGas1 = carrier gas\nGas2 = diluted gas\nArg = concentration"
        n131 = call <vilib>:"Clear Errors.vi"("error in (no error)"=w796) -> ("error out"=w790:errorcluster)  [unwired: 5 in, 1 out]
        n132 = case shown="False" w795 {
          tunnel: w803 -> [w809 w821]
          tunnel: [w809 w819] -> w802
          tunnel: w800 -> [w811 w818]
          tunnel: [w810 w817] -> w797
          tunnel: w794 -> [w808 w816]
          tunnel: [w807 w816] -> w793
          tunnel: [w806 w815] -> w788
          tunnel: w790 -> [w805 w814]
          tunnel: [w804 w813] -> w789
          frame True {
            n133 = call "TCP AK-LNI Befehl und Antwort.vi"("Fehler (Eingang)"=w805, "Sendedaten"=w811, "Befehl (4 Zeichen)"="EGAK", "Verbindungs-ID"=w808) -> ("Fehler (Ausgang)"=w810:errorcluster, "Empfangsdaten"=w806:string[], "Verbindungs-ID"=w807:refnum<k5>, "Befehl (Antwort)"=w804:string)  [unwired: 2 in, 2 out]
          }
          frame False {
            n134 = call "AK-LNI Befehl und Antwort.vi"("Fehler (Eingang)"=w814, "Sendedaten"=w818, "Befehl (4 Zeichen)"="EGAK", "VISA resource name"=w821) -> ("Fehler (Ausgang)"=w817:errorcluster, "Empfangsdaten"=w815:string[], "VISA resource name out"=w819:refnum<visa-resource-name>, "Befehl (Antwort)"=w813:string)  [unwired: 2 in, 2 out]
          }
        }
        n135 = Build Array (concatenate)(w789, w788) -> (w787:string[])
      }
      frame "AGAK" {
        # "Return the values of the set inlet gass\n\nBefehl:     AGAK K0\nAntwort:  AGAK ES Gas1 Gas2 Arg\n\nGas1 = carrier gas\nGas2 = diluted gas\nArg = concentration in ppm of the diluted gas"
        n136 = call <vilib>:"Clear Errors.vi"("error in (no error)"=w828) -> ("error out"=w822:errorcluster)  [unwired: 5 in, 1 out]
        n137 = case shown="False" w827 {
          tunnel: w835 -> [w837 w849]
          tunnel: [w837 w847] -> w834
          tunnel: [w841 w846] -> w830
          tunnel: [w840 w845] -> w829
          tunnel: w826 -> [w839 w844]
          tunnel: [w838 w844] -> w825
          tunnel: w822 -> [w836 w843]
          frame True {
            n138 = call "TCP AK-LNI Befehl und Antwort.vi"("Fehler (Eingang)"=w836, "Befehl (4 Zeichen)"="AGAK", "Verbindungs-ID"=w839) -> ("Fehler (Ausgang)"=w840:errorcluster, "Empfangsdaten"=w841:string[], "Verbindungs-ID"=w838:refnum<k5>)  [unwired: 3 in, 3 out]
          }
          frame False {
            n139 = call "AK-LNI Befehl und Antwort.vi"("Fehler (Eingang)"=w843, "Befehl (4 Zeichen)"="AGAK", "VISA resource name"=w849) -> ("Fehler (Ausgang)"=w845:errorcluster, "Empfangsdaten"=w846:string[], "VISA resource name out"=w847:refnum<visa-resource-name>)  [unwired: 3 in, 3 out]
          }
        }
      }
      frame "AKAK" {
        w862 = sgl 0.0  # SGL
        # "Return the final concentration in ppm of the selected dilution gas\n\nBefehl:     AKAK K0 [Point]\nAntwort:  AKAK K0 Point0 Dil1 Point2 Dil2 ..."
        n140 = call <vilib>:"Clear Errors.vi"("error in (no error)"=w857) -> ("error out"=w850:errorcluster)  [unwired: 5 in, 1 out]
        n141 = case shown="True" w855 {
          tunnel: w869 -> [w871 w885]
          tunnel: [w871 w883] -> w868
          tunnel: w866 -> [w876 w882]
          tunnel: [w875 w881] -> w858
          tunnel: [w874 w880] -> w856
          tunnel: w854 -> [w873 w879]
          tunnel: [w872 w879] -> w853
          tunnel: w850 -> [w870 w878]
          frame True {
            n142 = call "TCP AK-LNI Befehl und Antwort.vi"("Fehler (Eingang)"=w870, "Sendedaten"=w876, "Befehl (4 Zeichen)"="AKAK", "Verbindungs-ID"=w873) -> ("Fehler (Ausgang)"=w875:errorcluster, "Empfangsdaten"=w874:string[], "Verbindungs-ID"=w872:refnum<k5>)  [unwired: 2 in, 3 out]
          }
          frame False {
            n143 = call "AK-LNI Befehl und Antwort.vi"("Fehler (Eingang)"=w878, "Sendedaten"=w882, "Befehl (4 Zeichen)"="AKAK", "VISA resource name"=w885) -> ("Fehler (Ausgang)"=w881:errorcluster, "Empfangsdaten"=w880:string[], "VISA resource name out"=w883:refnum<visa-resource-name>)  [unwired: 2 in, 3 out]
          }
        }
        n144 = Index Array(array=w856, index=1 ("Index")) -> (element=w861:string)
        n145 = Fract/Exp String To Number(use system decimal point (T)=FALSE ("Systemdezimalzeichen verwenden (T)"), string=w861, default (0 dbl)=w862) -> (number=→"Konzentration":sgl)  [unwired: 1 in, 1 out]
      }
      frame "ALST" {
        # "Return the concentration in % of the selected dilution gas\n\nBefehl:     ALST K0 [Point]\nAntwort:  ALST K0 Point0 Dil1 Point2 Dil2 ..."
        n146 = call <vilib>:"Clear Errors.vi"("error in (no error)"=w893) -> ("error out"=w886:errorcluster)  [unwired: 5 in, 1 out]
        n147 = case shown="True" w891 {
          tunnel: w900 -> [w902 w916]
          tunnel: [w902 w914] -> w899
          tunnel: w897 -> [w907 w913]
          tunnel: [w906 w912] -> w894
          tunnel: [w905 w911] -> w892
          tunnel: w890 -> [w904 w910]
          tunnel: [w903 w910] -> w889
          tunnel: w886 -> [w901 w909]
          frame True {
            n148 = call "TCP AK-LNI Befehl und Antwort.vi"("Fehler (Eingang)"=w901, "Sendedaten"=w907, "Befehl (4 Zeichen)"="ALST", "Verbindungs-ID"=w904) -> ("Fehler (Ausgang)"=w906:errorcluster, "Empfangsdaten"=w905:string[], "Verbindungs-ID"=w903:refnum<k5>)  [unwired: 2 in, 3 out]
          }
          frame False {
            n149 = call "AK-LNI Befehl und Antwort.vi"("Fehler (Eingang)"=w909, "Sendedaten"=w913, "Befehl (4 Zeichen)"="ALST", "VISA resource name"=w916) -> ("Fehler (Ausgang)"=w912:errorcluster, "Empfangsdaten"=w911:string[], "VISA resource name out"=w914:refnum<visa-resource-name>)  [unwired: 2 in, 3 out]
          }
        }
      }
      frame "ADRU" {
        # "Druck-Rohwerte\n\nBefehl:     ADRU K0 [Line]\nAntwort:  ADRU ES Value1 Value2 Value3\n\nLine = 1  Read the pressure on the carrier line\nLine = 2  Read the pressure on the diluted line\nLine = 3  Read the output pressure (option)\nValue = The pressure of the corresponding Line"
        n150 = call <vilib>:"Clear Errors.vi"("error in (no error)"=w924) -> ("error out"=w917:errorcluster)  [unwired: 5 in, 1 out]
        n151 = case shown="False" w923 {
          tunnel: w931 -> [w934 w947]
          tunnel: [w934 w945] -> w930
          tunnel: w928 -> [w938 w944]
          tunnel: [w937 w943] -> w925
          tunnel: w922 -> [w936 w942]
          tunnel: [w935 w942] -> w921
          tunnel: [w933 w941] -> w918
          tunnel: w917 -> [w932 w940]
          frame True {
            n152 = call "TCP AK-LNI Befehl und Antwort.vi"("Fehler (Eingang)"=w932, "Sendedaten"=w938, "Befehl (4 Zeichen)"="ADRU", "Verbindungs-ID"=w936) -> ("Fehler (Ausgang)"=w937:errorcluster, "Empfangsdaten"=w933:string[], "Verbindungs-ID"=w935:refnum<k5>)  [unwired: 2 in, 3 out]
          }
          frame False {
            n153 = call "AK-LNI Befehl und Antwort.vi"("Fehler (Eingang)"=w940, "Sendedaten"=w944, "Befehl (4 Zeichen)"="ADRU", "VISA resource name"=w947) -> ("Fehler (Ausgang)"=w943:errorcluster, "Empfangsdaten"=w941:string[], "VISA resource name out"=w945:refnum<visa-resource-name>)  [unwired: 2 in, 3 out]
          }
        }
      }
      frame "SKOP" {
        # "Activate NOx converter tester\n\nBefehl:     SKOP K0 \nAntwort:  SKOP ES"
        n154 = call <vilib>:"Clear Errors.vi"("error in (no error)"=w957) -> ("error out"=w948:errorcluster)  [unwired: 5 in, 1 out]
        n155 = case shown="True" w956 {
          tunnel: w964 -> [w968 w982]
          tunnel: [w968 w980] -> w963
          tunnel: w961 -> [w972 w979]
          tunnel: [w971 w978] -> w958
          tunnel: w955 -> [w970 w977]
          tunnel: [w969 w977] -> w954
          tunnel: [w967 w976] -> w950
          tunnel: [w966 w975] -> w951
          tunnel: w948 -> [w965 w974]
          frame True {
            n156 = call "TCP AK-LNI Befehl und Antwort.vi"("Fehler (Eingang)"=w965, "Sendedaten"=w972, "Befehl (4 Zeichen)"="SKOP", "Verbindungs-ID"=w970) -> ("Fehler (Ausgang)"=w971:errorcluster, "Empfangsdaten"=w967:string[], "Verbindungs-ID"=w969:refnum<k5>, "Befehl (Antwort)"=w966:string)  [unwired: 2 in, 2 out]
          }
          frame False {
            n157 = call "AK-LNI Befehl und Antwort.vi"("Fehler (Eingang)"=w974, "Sendedaten"=w979, "Befehl (4 Zeichen)"="SKOP", "VISA resource name"=w982) -> ("Fehler (Ausgang)"=w978:errorcluster, "Empfangsdaten"=w976:string[], "VISA resource name out"=w980:refnum<visa-resource-name>, "Befehl (Antwort)"=w975:string)  [unwired: 2 in, 2 out]
          }
        }
        n158 = Build Array (concatenate)(w951, w950) -> (w949:string[])
      }
      frame "SVIO" {
        # "SVIO Select the desired diluted\ninlet (if the option is\ninstalled).\nsent: + SVIO K0 13+\nreceived: + SVIO 0"
        n159 = call <vilib>:"Clear Errors.vi"("error in (no error)"=w990) -> ("error out"=w983:errorcluster)  [unwired: 5 in, 1 out]
        n160 = case shown="True" w989 {
          tunnel: w997 -> [w1002 w1017]
          tunnel: [w1002 w1015] -> w996
          tunnel: w994 -> [w1006 w1014]
          tunnel: [w1005 w1013] -> w991
          tunnel: w988 -> [w1004 w1012]
          tunnel: [w1003 w1012] -> w987
          tunnel: [w999 w1009] -> w984
          tunnel: w983 -> [w998 w1008]
          frame True {
            n161 = call "TCP AK-LNI Befehl und Antwort.vi"("Fehler (Eingang)"=w998, "Sendedaten"=w1006, "Befehl (4 Zeichen)"="SVIO", "Verbindungs-ID"=w1004) -> ("Fehler (Ausgang)"=w1005:errorcluster, "Empfangsdaten"=w1000:string[], "Verbindungs-ID"=w1003:refnum<k5>, "Befehl (Antwort)"=w1001:string)  [unwired: 2 in, 2 out]
            n162 = Build Array (concatenate)(w1001, w1000) -> (w999:string[])
          }
          frame False {
            n163 = call "AK-LNI Befehl und Antwort.vi"("Fehler (Eingang)"=w1008, "Sendedaten"=w1014, "Befehl (4 Zeichen)"="SVIO", "VISA resource name"=w1017) -> ("Fehler (Ausgang)"=w1013:errorcluster, "Empfangsdaten"=w1010:string[], "VISA resource name out"=w1015:refnum<visa-resource-name>, "Befehl (Antwort)"=w1011:string)  [unwired: 2 in, 2 out]
            n164 = Build Array (concatenate)(w1011, w1010) -> (w1009:string[])
          }
        }
      }
      frame "SVSA" {
        # "Open functions for the NOX converter tester\n\nBefehl:     SVSA K0 Arg\nAntwort:  SVSA ES\n\nArg = 101   generate ozone\nArg = 102   switch on the AIR valve (like SAIR)\nArg = 103   switch on the NO valve (like SONO)"
        n165 = call <vilib>:"Clear Errors.vi"("error in (no error)"=w1018) -> ()  [unwired: 5 in, 2 out]
        n166 = case shown="False" w1026 {
          tunnel: w1033 -> [w1037 w1051]
          tunnel: [w1037 w1049] -> w1032
          tunnel: w1030 -> [w1041 w1048]
          tunnel: [w1040 w1047] -> w1027
          tunnel: w1025 -> [w1039 w1046]
          tunnel: [w1038 w1046] -> w1024
          tunnel: [w1036 w1044] -> w1020
          tunnel: [w1035 w1045] -> w1021
          tunnel: w1018 -> [w1034 w1043]
          frame True {
            n167 = call "TCP AK-LNI Befehl und Antwort.vi"("Fehler (Eingang)"=w1034, "Sendedaten"=w1041, "Befehl (4 Zeichen)"="SVSA", "Verbindungs-ID"=w1039) -> ("Fehler (Ausgang)"=w1040:errorcluster, "Empfangsdaten"=w1036:string[], "Verbindungs-ID"=w1038:refnum<k5>, "Befehl (Antwort)"=w1035:string)  [unwired: 2 in, 2 out]
          }
          frame False {
            n168 = call "AK-LNI Befehl und Antwort.vi"("Fehler (Eingang)"=w1043, "Sendedaten"=w1048, "Befehl (4 Zeichen)"="SVSA", "VISA resource name"=w1051) -> ("Fehler (Ausgang)"=w1047:errorcluster, "Empfangsdaten"=w1044:string[], "VISA resource name out"=w1049:refnum<visa-resource-name>, "Befehl (Antwort)"=w1045:string)  [unwired: 2 in, 2 out]
          }
        }
        n169 = Build Array (concatenate)(w1021, w1020) -> (w1019:string[])
      }
      frame "SVSZ" {
        # "Close functions for the NOX converter tester\n\nBefehl:     SVSZ K0 Arg\nAntwort:  SVSZ ES\n\nArg = 101   stop the ozone\nArg = 102   switch off the AIR valve (like SAIR)\nArg = 103   switch off the NO valve (like SONO)"
        n170 = call <vilib>:"Clear Errors.vi"("error in (no error)"=w1061) -> ("error out"=w1052:errorcluster)  [unwired: 5 in, 1 out]
        n171 = case shown="False" w1060 {
          tunnel: w1068 -> [w1072 w1086]
          tunnel: [w1072 w1084] -> w1067
          tunnel: w1065 -> [w1076 w1083]
          tunnel: [w1075 w1082] -> w1062
          tunnel: w1059 -> [w1074 w1081]
          tunnel: [w1073 w1081] -> w1058
          tunnel: [w1070 w1080] -> w1054
          tunnel: [w1071 w1079] -> w1055
          tunnel: w1052 -> [w1069 w1078]
          frame True {
            n172 = call "TCP AK-LNI Befehl und Antwort.vi"("Fehler (Eingang)"=w1069, "Sendedaten"=w1076, "Befehl (4 Zeichen)"="SVSZ", "Verbindungs-ID"=w1074) -> ("Fehler (Ausgang)"=w1075:errorcluster, "Empfangsdaten"=w1070:string[], "Verbindungs-ID"=w1073:refnum<k5>, "Befehl (Antwort)"=w1071:string)  [unwired: 2 in, 2 out]
          }
          frame False {
            n173 = call "AK-LNI Befehl und Antwort.vi"("Fehler (Eingang)"=w1078, "Sendedaten"=w1083, "Befehl (4 Zeichen)"="SVSZ", "VISA resource name"=w1086) -> ("Fehler (Ausgang)"=w1082:errorcluster, "Empfangsdaten"=w1080:string[], "VISA resource name out"=w1084:refnum<visa-resource-name>, "Befehl (Antwort)"=w1079:string)  [unwired: 2 in, 2 out]
          }
        }
        n174 = Build Array (concatenate)(w1055, w1054) -> (w1053:string[])
      }
      frame "SONO" {
        # "Open or close the valves in order to perform the NO phase \nof the NOx converter tester\n\nBefehl:     SONO K0 Arg\nAntwort:  SONO ES\n\nArg = 1   Open the valves\nArg = 0   Close the valves"
        n175 = call <vilib>:"Clear Errors.vi"("error in (no error)"=w1096) -> ("error out"=w1087:errorcluster)  [unwired: 5 in, 1 out]
        n176 = case shown="True" w1095 {
          tunnel: w1103 -> [w1107 w1121]
          tunnel: [w1107 w1119] -> w1102
          tunnel: w1100 -> [w1111 w1118]
          tunnel: [w1110 w1117] -> w1097
          tunnel: w1094 -> [w1109 w1116]
          tunnel: [w1108 w1116] -> w1093
          tunnel: [w1106 w1115] -> w1089
          tunnel: [w1105 w1114] -> w1090
          tunnel: w1087 -> [w1104 w1113]
          frame True {
            n177 = call "TCP AK-LNI Befehl und Antwort.vi"("Fehler (Eingang)"=w1104, "Sendedaten"=w1111, "Befehl (4 Zeichen)"="SONO", "Verbindungs-ID"=w1109) -> ("Fehler (Ausgang)"=w1110:errorcluster, "Empfangsdaten"=w1106:string[], "Verbindungs-ID"=w1108:refnum<k5>, "Befehl (Antwort)"=w1105:string)  [unwired: 2 in, 2 out]
          }
          frame False {
            n178 = call "AK-LNI Befehl und Antwort.vi"("Fehler (Eingang)"=w1113, "Sendedaten"=w1118, "Befehl (4 Zeichen)"="SONO", "VISA resource name"=w1121) -> ("Fehler (Ausgang)"=w1117:errorcluster, "Empfangsdaten"=w1115:string[], "VISA resource name out"=w1119:refnum<visa-resource-name>, "Befehl (Antwort)"=w1114:string)  [unwired: 2 in, 2 out]
          }
        }
        n179 = Build Array (concatenate)(w1090, w1089) -> (w1088:string[])
      }
      frame "SAIR" {
        # "Open or close the valves in order to perform the Air phase \nof the NOx converter tester\n\nBefehl:     SAIR K0 Arg\nAntwort:  SAIR ES\n\nArg = 1   Open the valves\nArg = 0   Close the valves"
        n180 = call <vilib>:"Clear Errors.vi"("error in (no error)"=w1131) -> ("error out"=w1122:errorcluster)  [unwired: 5 in, 1 out]
        n181 = case shown="False" w1130 {
          tunnel: w1138 -> [w1142 w1156]
          tunnel: [w1142 w1154] -> w1137
          tunnel: w1135 -> [w1146 w1153]
          tunnel: [w1145 w1152] -> w1132
          tunnel: w1129 -> [w1144 w1151]
          tunnel: [w1143 w1151] -> w1128
          tunnel: [w1141 w1150] -> w1124
          tunnel: [w1140 w1149] -> w1125
          tunnel: w1122 -> [w1139 w1148]
          frame True {
            n182 = call "TCP AK-LNI Befehl und Antwort.vi"("Fehler (Eingang)"=w1139, "Sendedaten"=w1146, "Befehl (4 Zeichen)"="SAIR", "Verbindungs-ID"=w1144) -> ("Fehler (Ausgang)"=w1145:errorcluster, "Empfangsdaten"=w1141:string[], "Verbindungs-ID"=w1143:refnum<k5>, "Befehl (Antwort)"=w1140:string)  [unwired: 2 in, 2 out]
          }
          frame False {
            n183 = call "AK-LNI Befehl und Antwort.vi"("Fehler (Eingang)"=w1148, "Sendedaten"=w1153, "Befehl (4 Zeichen)"="SAIR", "VISA resource name"=w1156) -> ("Fehler (Ausgang)"=w1152:errorcluster, "Empfangsdaten"=w1150:string[], "VISA resource name out"=w1154:refnum<visa-resource-name>, "Befehl (Antwort)"=w1149:string)  [unwired: 2 in, 2 out]
          }
        }
        n184 = Build Array (concatenate)(w1125, w1124) -> (w1123:string[])
      }
      frame "SNOX" {
        # "Set the ozone in order to generate NO2 phase of the NOX converter tester\nPay attention: the commands SONO and SAIR must have been sent previously \n\n\nBefehl:     SNOX K0 Arg\nAntwort:  SNOX ES\n\nArg = desired NO2 value (0 = minimal and 100 = maximal value)"
        n185 = call <vilib>:"Clear Errors.vi"("error in (no error)"=w1166) -> ("error out"=w1157:errorcluster)  [unwired: 5 in, 1 out]
        n186 = case shown="True" w1165 {
          tunnel: w1173 -> [w1177 w1191]
          tunnel: [w1177 w1189] -> w1172
          tunnel: w1170 -> [w1181 w1188]
          tunnel: [w1180 w1187] -> w1167
          tunnel: w1164 -> [w1179 w1186]
          tunnel: [w1178 w1186] -> w1163
          tunnel: [w1176 w1185] -> w1159
          tunnel: [w1175 w1184] -> w1160
          tunnel: w1157 -> [w1174 w1183]
          frame True {
            n187 = call "TCP AK-LNI Befehl und Antwort.vi"("Fehler (Eingang)"=w1174, "Sendedaten"=w1181, "Befehl (4 Zeichen)"="SNOX", "Verbindungs-ID"=w1179) -> ("Fehler (Ausgang)"=w1180:errorcluster, "Empfangsdaten"=w1176:string[], "Verbindungs-ID"=w1178:refnum<k5>, "Befehl (Antwort)"=w1175:string)  [unwired: 2 in, 2 out]
          }
          frame False {
            n188 = call "AK-LNI Befehl und Antwort.vi"("Fehler (Eingang)"=w1183, "Sendedaten"=w1188, "Befehl (4 Zeichen)"="SNOX", "VISA resource name"=w1191) -> ("Fehler (Ausgang)"=w1187:errorcluster, "Empfangsdaten"=w1185:string[], "VISA resource name out"=w1189:refnum<visa-resource-name>, "Befehl (Antwort)"=w1184:string)  [unwired: 2 in, 2 out]
          }
        }
        n189 = Build Array (concatenate)(w1160, w1159) -> (w1158:string[])
      }
      frame "ANOX" {
        w1203 = sgl 0.0  # SGL
        # "Read the set ozone value \n\nBefehl:     ANOX K0\nAntwort:  SNOX ES Arg\n\nArg = desired NO2 value (0 = minimal and 100 = maximal value)"
        n190 = call <vilib>:"Clear Errors.vi"("error in (no error)"=w1199) -> ("error out"=w1192:errorcluster)  [unwired: 5 in, 1 out]
        n191 = case shown="False" w1198 {
          tunnel: w1210 -> [w1212 w1226]
          tunnel: [w1212 w1224] -> w1209
          tunnel: w1207 -> [w1217 w1223]
          tunnel: [w1216 w1222] -> w1193
          tunnel: [w1215 w1221] -> w1200
          tunnel: w1197 -> [w1214 w1220]
          tunnel: [w1213 w1220] -> w1196
          tunnel: w1192 -> [w1211 w1219]
          frame True {
            n192 = call "TCP AK-LNI Befehl und Antwort.vi"("Fehler (Eingang)"=w1211, "Sendedaten"=w1217, "Befehl (4 Zeichen)"="ANOX", "Verbindungs-ID"=w1214) -> ("Fehler (Ausgang)"=w1215:errorcluster, "Empfangsdaten"=w1216:string[], "Verbindungs-ID"=w1213:refnum<k5>)  [unwired: 2 in, 3 out]
          }
          frame False {
            n193 = call "AK-LNI Befehl und Antwort.vi"("Fehler (Eingang)"=w1219, "Sendedaten"=w1223, "Befehl (4 Zeichen)"="ANOX", "VISA resource name"=w1226) -> ("Fehler (Ausgang)"=w1221:errorcluster, "Empfangsdaten"=w1222:string[], "VISA resource name out"=w1224:refnum<visa-resource-name>)  [unwired: 2 in, 3 out]
          }
        }
        n194 = Index Array(array=w1193) -> (element=w1202:string)  [unwired: 1 in]
        n195 = Fract/Exp String To Number(use system decimal point (T)=FALSE ("Systemdezimalzeichen verwenden (T)"), string=w1202, default (0 dbl)=w1203) -> (number=w1201:sgl)  [unwired: 1 in, 1 out]
        n196 = local write "Konzentration"(w1201) -> ()
      }
    }
  }
  "Status" <- w7
  "Empfangsdaten" <- w6
  "Verfügbare Gase" <- w5
  "Error" <- w4
  "Betriebsart" <- w1
  n197 = Unbundle By Name(w3) -> ("status"=→"Störung Kommunikation":bool)
